vi "Clear Buffer.vi"(8 "error in (no error)":errorcluster, 10 "Buffer Name (\"\")":string, 11 "VISA resource name":refnum<visa-resource-name>) -> (0 "error out":errorcluster, 3 "VISA resource name out":refnum<visa-resource-name>)   [LabVIEW 2024, in "Keithley DMM6500 DAQ6500 Series.lvlib"]
doc: "Clears the buffer specified by \"Buffer Name\""
uses:
  Keithley DMM6500 DAQ6500 Series.lvlib
  <vilib>/Utility/error.llb/Trim Whitespace One-Sided.vi
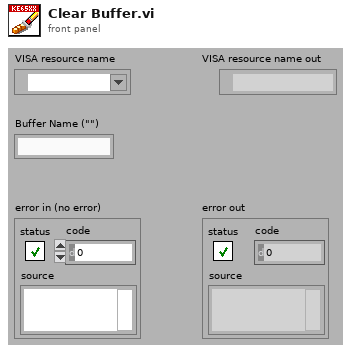
[diagram p1: front panel]
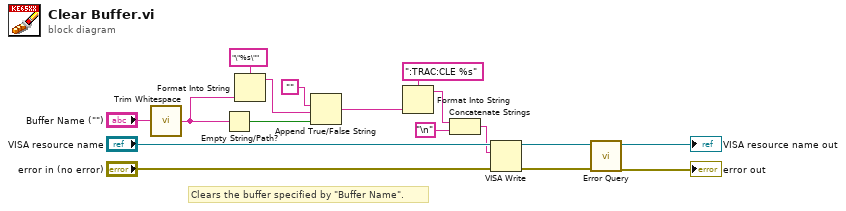
[diagram p0: block diagram]
diagram:
  # "Clears the buffer specified by \"Buffer Name\"."
  n1 = call <vilib>:"Trim Whitespace.vi"("string"="Buffer Name (\"\")") -> ("trimmed string"=w2:string)  [unwired: 1 in]
  n2 = Empty String/Path?(string/path=w2) -> (empty?=w1:bool)
  n3 = Format Into String(format string="\"%s\"", w2) -> (resulting string=w4:string)  [unwired: 2 in, 1 out]
  n4 = Append True/False String(1:w1, 2:w4, 3:"") -> (0:w6:string)  [unwired: 1 in]
  n5 = Format Into String(format string=":TRAC:CLE %s", w6) -> (resulting string=w7:string)  [unwired: 2 in, 1 out]
  n6 = Concatenate Strings(w7, "\n") -> (w10:string)
  n7 = VISA Write(VISA resource name="VISA resource name", write buffer=w10, error in (no error)="error in (no error)") -> (VISA resource name out=w14:refnum<visa-resource-name>, error out=w13:errorcluster)  [unwired: 1 out]
  n8 = call "Error Query.vi"("error in (no error)"=w13, "VISA resource name"=w14) -> ("error out"=→"error out":errorcluster, "VISA resource name out"=→"VISA resource name out":refnum<visa-resource-name>)  [unwired: 6 in, 2 out]
